vi "2 Speed Auto Shifter.vi"(5 "Enable":bool, 7 "Down Shift Value":dbl, 8 "Up Shift Value":dbl, 9 "Right Enc Rate":dbl, 10 "Left  Enc Rate":dbl) -> (0 "Down Shift":bool, 3 "Up Shift":bool)   [LabVIEW 2014]
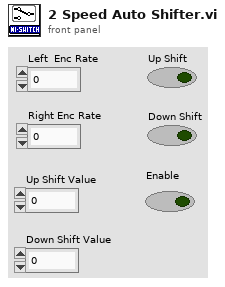
[diagram p1: front panel]
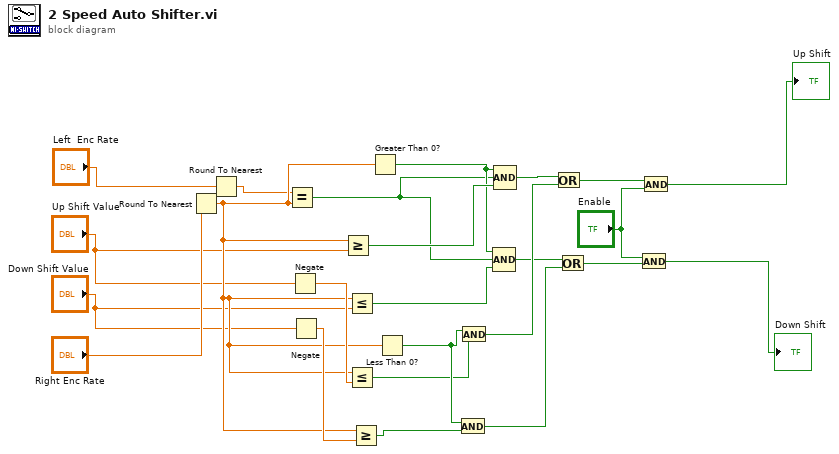
[diagram p0: block diagram]
diagram:
  n1 = Round To Nearest(number="Right Enc Rate") -> (nearest integer value=w17:dbl)
  n2 = Round To Nearest(number="Left  Enc Rate") -> (nearest integer value=w14:dbl)
  n3 = Equal?(x=w14, y=w17) -> (x = y?=w2:bool)
  n4 = Negate(x="Up Shift Value") -> (-x=w23:dbl)
  n5 = Negate(x="Down Shift Value") -> (-x=w24:dbl)
  n6 = Greater Or Equal?(x=w17, y="Up Shift Value") -> (x >= y?=w5:bool)
  n7 = Less Or Equal?(x=w17, y="Down Shift Value") -> (x <= y?=w1:bool)
  n8 = Less Or Equal?(x=w17, y=w23) -> (x <= y?=w19:bool)
  n9 = Greater Or Equal?(x=w17, y=w24) -> (x >= y?=w22:bool)
  n10 = Greater Than 0?(x=w17) -> (x > 0?=w3:bool)
  n11 = Less Than 0?(x=w17) -> (x < 0?=w20:bool)
  n12 = And(x=w20, y=w22) -> (x .and. y?=w21:bool)
  n13 = And(x=w20, y=w19) -> (x .and. y?=w18:bool)
  n14 = Compound Arithmetic op=AND(w3, w2, w1) -> (w4:bool)
  n15 = Compound Arithmetic op=AND(w3, w2, w5) -> (w6:bool)
  n16 = Or(x=w6, y=w18) -> (x .or. y?=w9:bool)
  n17 = Or(x=w4, y=w21) -> (x .or. y?=w8:bool)
  n18 = And(x="Enable", y=w8) -> (x .and. y?=→"Down Shift":bool)
  n19 = And(x=w9, y="Enable") -> (x .and. y?=→"Up Shift":bool)
